vi "Create New File.vi"(8 "error in (no error)":errorcluster, 11 "file handler in":refnum<class "File Handler.lvclass">) -> (0 "error out":errorcluster, 3 "file handler out":refnum<class "File Handler.lvclass">)   [LabVIEW 2018, in "GLog.lvlib" / "File Handler.lvclass"]
uses:
  File Handler.lvclass
  File Handler.lvclass/File Handler.ctl
panel:
  # "Connector Pane"
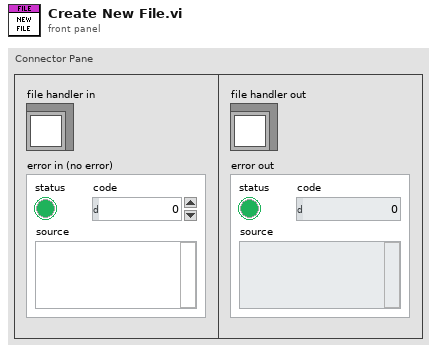
[diagram p1: front panel]
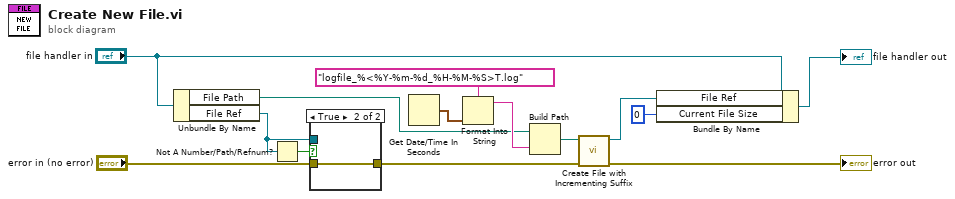
[diagram p0: block diagram]
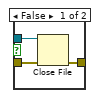
[diagram p2: hidden frame]
diagram:
  n1 = Unbundle By Name("file handler in") -> ("File Path"=w8:path, "File Ref"=w2:refnum<file>)
  n2 = Not A Number/Path/Refnum?(number/path/refnum=w2) -> (NaN/Path/Refnum?=w1:bool)
  n3 = case shown="True" w1 {
    tunnel: "error in (no error)" -> [w17 w18]
    tunnel: [w16 w18] -> w3
    tunnel: w2 -> [w15 _]
    frame False {
      n4 = Close File(refnum=w15, error in=w17) -> (error out=w16:errorcluster)  [unwired: 1 out]
    }
    frame True {
    }
  }
  n5 = Get Date/Time In Seconds() -> (seconds since 1Jan1904=w14:timestamp)
  n6 = Format Into String(format string="logfile_%<%Y-%m-%d_%H-%M-%S>T.log", w14) -> (resulting string=w13:string)  [unwired: 2 in, 1 out]
  n7 = Build Path(base path=w8, name or relative path=w13) -> (appended path=w7:path)
  n8 = call <vilib>:"Create File with Incrementing Suffix.vi"("error in (no error)"=w3, "file path"=w7) -> ("error out"=→"error out":errorcluster, "refnum out"=w4:refnum<file>)  [unwired: 7 in, 1 out]
  n9 = Bundle By Name(cluster="file handler in", "File Ref"=w4, "Current File Size"=u64 0) -> (→"file handler out":refnum<class "File Handler.lvclass">)
